vi "Parse.vi"(8 "error in":errorcluster, 11 "MessageStr":string) -> (0 "error out":errorcluster, 2 "MessageVar":variant, 3 "MessageType":T1)   [LabVIEW 2020, in "NMEA.lvlib"]
uses:
  NMEA.lvlib
  NMEA_GPVTG-data.ctl
  NMEA_Mode.ctl
  NMEA_GPRMC-data.ctl
  NMEA_LatitudeDirection.ctl
  NMEA_LongitudeDirection.ctl
  NMEA_GPGGA-data.ctl
  NMEA_GPS-Quality.ctl
  NMEA_Type.ctl
panel:
  out "$GPGGA-message_OUT":T2={"TimeStamp"=timestamp(0 s since 1904-01-01), "Latitude"=0.0, "Latitude-Direction"=enum."", "Longitude"=1.0, "Longitude-Direction"=enum."", "GPS-Quality"=enum."GPS fix (SPS)", "Number of Satellites"=0, "Horizontal Dilution of Precision"=0.0, "Altitude above Mean-Sea-Level"=0.0, "Geoidal separation"=0.0, "Time since last DGPS update"=0.0, "DGPS reference station ID"=0} {"Time since last DGPS update" format="%.02f [s]"; "Geoidal separation" format="%.02f [m]"; "Altitude above Mean-Sea-Level" format="%.02f [m]"; "Horizontal Dilution of Precision" format="%.02f [HDOP]"; "Longitude" format="%0.4f [long]"; "Latitude" format="%.04f [lat]"; "TimeStamp" format="%<%.2X>T"}
  out "TX LAT":dbl
  out "TX LONG":dbl
  out "Data":string[][](table)
  out "$GPRMC-message_OUT":T6={"TimeStamp"=timestamp(0 s since 1904-01-01), "Validity"=FALSE, "Latitude"=0.0, "Latitude-Direction"=enum."North", "Longitude"=0.0, "Longitude-Direction"=enum."East", "Speed in knots"=0.0, "True course"=0.0, "Date Stamp"=timestamp(0 s since 1904-01-01), "Magnetic Variation (East/West)"=0.0} {"Magnetic Variation (East/West)" format="%.02f [deg]"; "Date Stamp" format="%<%x>T"; "True course" format="%.02f [deg]"; "Speed in knots" format="%.02f [kts]"; "Longitude" format="%0.4f [long]"; "Latitude" format="%.04f [lat]"; "TimeStamp" format="%<%.2X>T"}
  out "$GPVTG-message_OUT":T7={"True Course over Ground"=0.0, "Magnetic Course over Ground"=0.0, "Speed over Ground in knots"=0.0, "Speed over Ground in km/h"=1.0, "Mode"=""} {"Speed over Ground in km/h" format="%.02f [km/h]"; "Speed over Ground in knots" format="%.02f [kts]"; "Magnetic Course over Ground" format="%.02f [deg]"; "True Course over Ground" format="%.02f [deg]"}
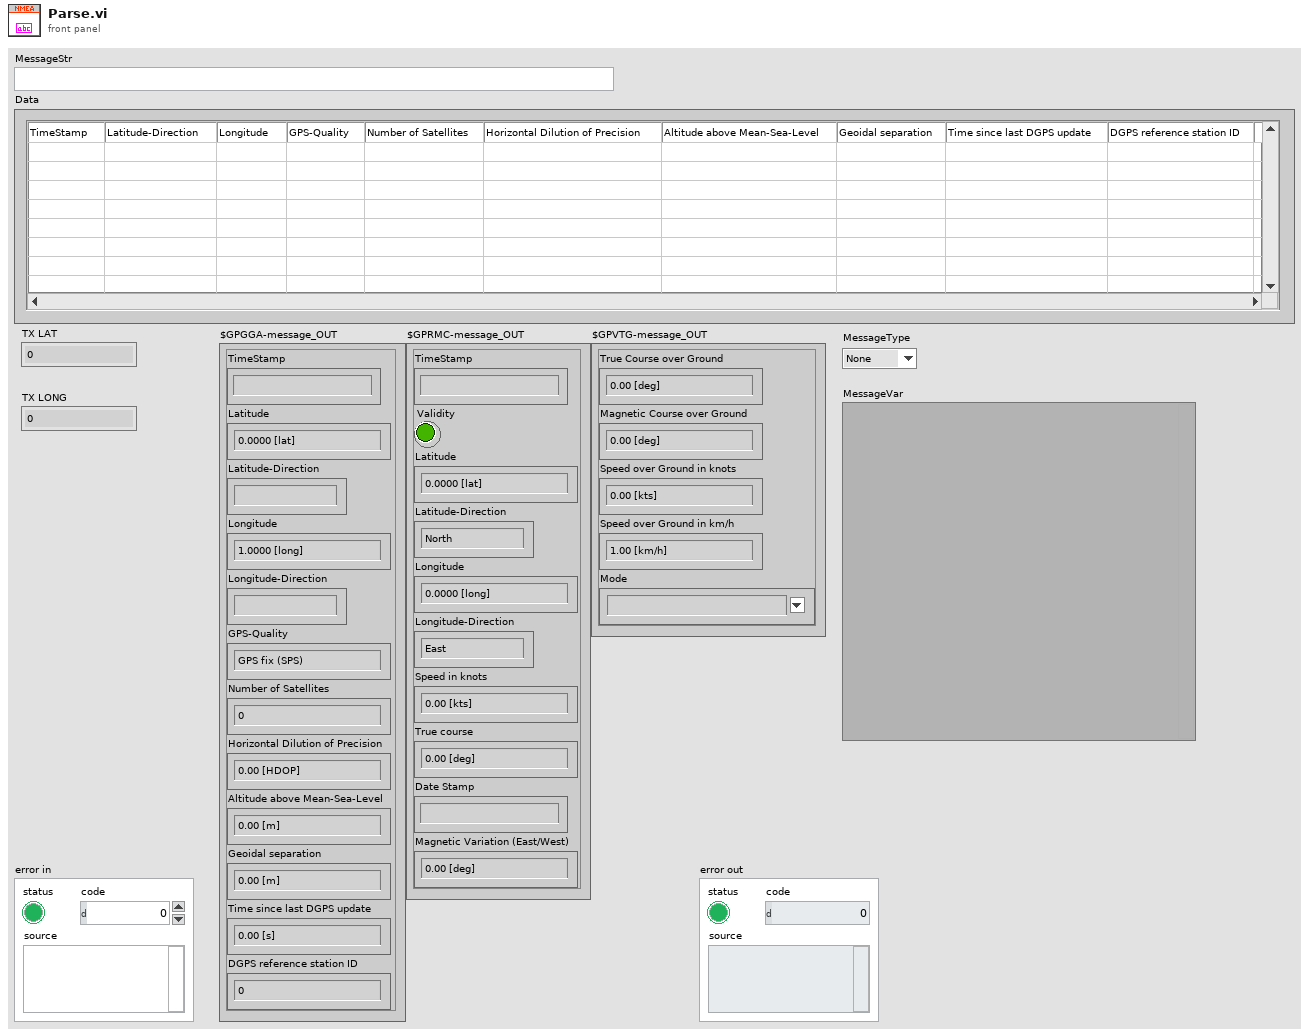
[diagram p1: front panel]
types:
  T1 = typedef "NMEA.lvlib/NMEA_Type.ctl" = enum16{"None", "GGA", "VTG", "RMC"}
  T2 = typedef "NMEA.lvlib/NMEA_GPGGA-data.ctl" = cluster{"TimeStamp":timestamp, "Latitude":dbl, "Latitude-Direction":T3, "Longitude":dbl, "Longitude-Direction":T4, "GPS-Quality":T5, "Number of Satellites":i32, "Horizontal Dilution of Precision":dbl, "Altitude above Mean-Sea-Level":dbl, "Geoidal separation":dbl, "Time since last DGPS update":dbl, "DGPS reference station ID":i32}
  T3 = typedef "NMEA.lvlib/NMEA_LatitudeDirection.ctl" = enum16{"", "North", "South"}
  T4 = typedef "NMEA.lvlib/NMEA_LongitudeDirection.ctl" = enum16{"", "East", "West"}
  T5 = typedef "NMEA.lvlib/NMEA_GPS-Quality.ctl" = enum16{"Invalid", "GPS fix (SPS)", "DGPS fix", "PPS fix", "Real Time Kinematic", "Float RTK", "estimated", "Manual input mode", "Simulation mode"}
  T6 = typedef "NMEA.lvlib/NMEA_GPRMC-data.ctl" = cluster{"TimeStamp":timestamp, "Validity":bool, "Latitude":dbl, "Latitude-Direction":T3, "Longitude":dbl, "Longitude-Direction":T4, "Speed in knots":dbl, "True course":dbl, "Date Stamp":timestamp, "Magnetic Variation (East/West)":dbl}
  T7 = typedef "NMEA.lvlib/NMEA_GPVTG-data.ctl" = cluster{"True Course over Ground":dbl, "Magnetic Course over Ground":dbl, "Speed over Ground in knots":dbl, "Speed over Ground in km/h":dbl, "Mode":T8}
  T8 = typedef "NMEA.lvlib/NMEA_Mode.ctl" = string
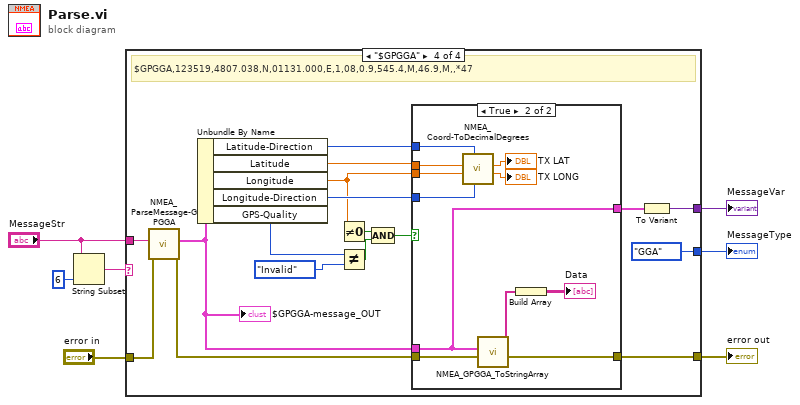
[diagram p0: block diagram]
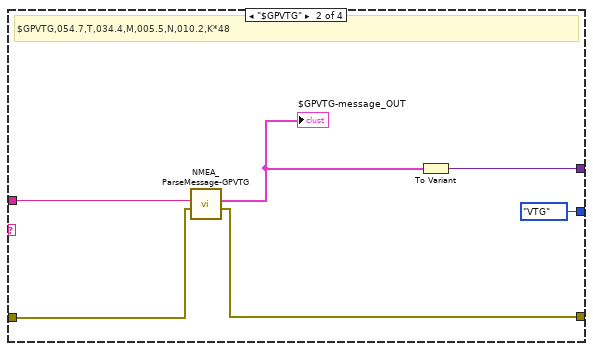
[diagram p3: hidden frame]
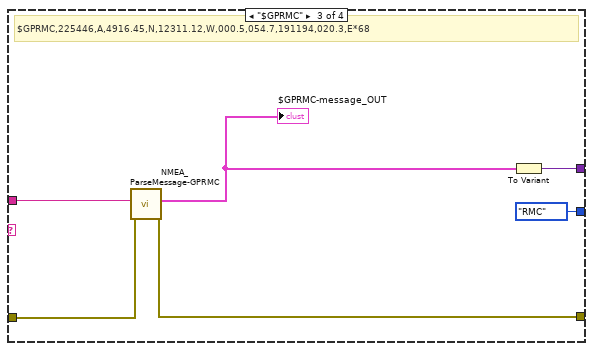
[diagram p4: hidden frame]
diagram:
  n1 = String Subset(string="MessageStr", length (rest)=6 ("longueur (reste)")) -> (substring=w6:string)  [unwired: 1 in]
  n2 = case "Handling NMEA Frames" shown="\"$GPGGA\"" w6 {
    tunnel: "MessageStr" -> [_ w14 w20 w37]
    tunnel: "error in" -> [w8 w13 w19 w25]
    tunnel: [w8 w12 w18 w24] -> w3
    tunnel: [_ NMEA_Type."VTG" ("MessageType") NMEA_Type."RMC" ("MessageType") NMEA_Type."GGA" ("MessageType")] -> w2
    tunnel: [_ w10 w16 w21] -> w1
    frame " ", Default {
    }
    frame "$GPVTG" {
      # "$GPVTG,054.7,T,034.4,M,005.5,N,010.2,K*48"
      n3 = call "NMEA_ParseMessage-GPVTG.vi"("Error In"=w13, "$GPVTG-message_IN"=w14) -> ("Error Out"=w12:errorcluster, "$GPVTG-message_OUT"=w11:T7)  [unwired: 8 in]
      "$GPVTG-message_OUT" <- w11
      n4 = To Variant(anything=w11) -> (Variant=w10:variant)
    }
    frame "$GPRMC" {
      # "$GPRMC,225446,A,4916.45,N,12311.12,W,000.5,054.7,191194,020.3,E*68"
      n5 = call "NMEA_ParseMessage-GPRMC.vi"("Error In"=w19, "$GPRMC-message_IN"=w20) -> ("Error Out"=w18:errorcluster, "$GPRMC-message_OUT"=w17:T6)  [unwired: 8 in]
      "$GPRMC-message_OUT" <- w17
      n6 = To Variant(anything=w17) -> (Variant=w16:variant)
    }
    frame "$GPGGA" {
      # "$GPGGA,123519,4807.038,N,01131.000,E,1,08,0.9,545.4,M,46.9,M,,*47"
      n7 = call "NMEA_ParseMessage-GPGGA.vi"("Error In"=w25, "$GPGGA-message_IN"=w37) -> ("Error Out"=w26:errorcluster, "$GPGGA-message_OUT"=w33:T2)  [unwired: 8 in]
      "$GPGGA-message_OUT" <- w33
      n8 = Unbundle By Name(w33) -> ("Latitude-Direction"=w34:T3, "Latitude"=w35:dbl, "Longitude"=w32:dbl, "Longitude-Direction"=w36:T4, "GPS-Quality"=w27:T5)
      n9 = Not Equal To 0?(x=w32) -> (x != 0?=w30:bool)
      n10 = Not Equal?(x=w27, y=NMEA_GPS-Quality."Invalid" ("GPS-Quality")) -> (x != y?=w28:bool)
      n11 = Compound Arithmetic op=AND(w30, w28) -> (w31:bool)
      n12 = case shown="True" w31 {
        tunnel: w36 -> [_ w47]
        tunnel: w35 -> [_ w44]
        tunnel: w34 -> [_ w43]
        tunnel: w33 -> [_ w39]
        tunnel: w32 -> [_ w45]
        tunnel: w26 -> [w38 w42]
        tunnel: [w38 w41] -> w24
        tunnel: [_ w39] -> w22
        frame False {
        }
        frame True {
          n13 = call "NMEA_Coord-ToDecimalDegrees.vi"("Longitude-Direction"=w47, "Latitude-Direction"=w43, "Longitude"=w45, "Latitude"=w44) -> ("Longitude"=→"TX LONG":dbl, "Latitude"=→"TX LAT":dbl)  [unwired: 6 in]
          n14 = call "NMEA_GPGGA_ToStringArray.vi"("Error In"=w42, "$GPGGA-message_IN"=w39) -> ("Error Out"=w41:errorcluster, "$GPGGA-message_OUT"=w46:string[])  [unwired: 8 in]
          n15 = Build Array(w46) -> (→"Data":string[][])
        }
      }
      n16 = To Variant(anything=w22) -> (Variant=w21:variant)
    }
  }
  "error out" <- w3
  "MessageVar" <- w1
  "MessageType" <- w2
